vi "Copy Value.vi"(10 "From":refnum<class "Type.lvclass">, 11 "Timestamp in":refnum<class "Timestamp.lvclass">) -> (2 "error out":errorcluster, 3 "Timestamp out":refnum<class "Timestamp.lvclass">)   [LabVIEW 2020, in "Conditu2.lvlib" / "Columns.lvlib" / "Timestamp.lvclass"]
uses:
  Timestamp.lvclass
  C:/dev/lv20CE/lv-conditum-tools/Conditum-Clone/Columns/Type/Type.lvclass
  Type/Type.lvclass
  Timestamp.lvclass/Timestamp.ctl
  Type/Type.lvclass/Type.ctl
  Type/Clear NULL.vi
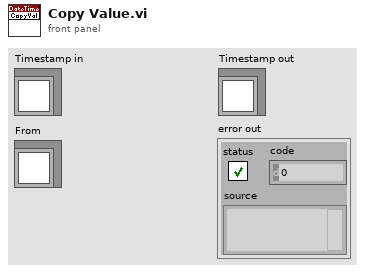
[diagram p1: front panel]
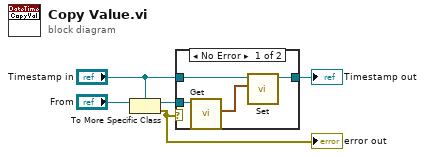
[diagram p0: block diagram]
diagram:
  n1 = To More Specific Class(target class="Timestamp in", reference="From") -> (specific class reference=w5:refnum<class "Timestamp.lvclass">, error out=w3:errorcluster)  [unwired: 1 in]
  "error out" <- w3
  n2 = case shown="No Error" w3 {
    tunnel: w5 -> [w9 _]
    tunnel: "Timestamp in" -> [w7 w10]
    tunnel: [w6 w10] -> w4
    frame No Error {
      n3 = call "Get.vi"("Timestamp in"=w9) -> ("Value"=w8:timestamp)  [unwired: 10 in]
      n4 = call "Set.vi"("Time Stamp"=w8, "DateTime in"=w7) -> ("DateTime out"=w6:refnum<class "Timestamp.lvclass">)  [unwired: 9 in]
    }
    frame Error {
    }
  }
  "Timestamp out" <- w4
